vi "write module trace msg.vi"(8 "error in (no error)":errorcluster, 9 "Priority":T1(ring)=enum."Debug", 10 "message":string, 11 "module in":refnum<class "TBM module execution interface.lvclass">) -> (0 "error out":errorcluster, 3 "module out":refnum<class "TBM module execution interface.lvclass">)   [LabVIEW 2013, in "TBM module execution interface.lvclass"]
uses:
  TBM module execution interface.lvclass
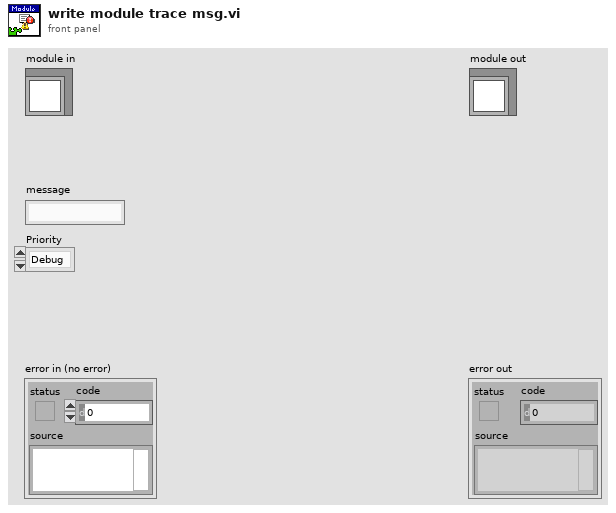
[diagram p1: front panel]
types:
  T1 = enum16{"Emergency", "Alert", "Critical", "Error", "Warning", "Notice", "Informational", "Debug"}
  T2 = enum16{"kern", "user", "mail", "daemon", "auth", "syslog", "lpr", "news", "uucp", "clk", "authpriv", "ftp", "NTP", "log audit", "log alert", "cron", "local0", "local1", "local2", "local3", "local4", "local5", "local6", "local7"}
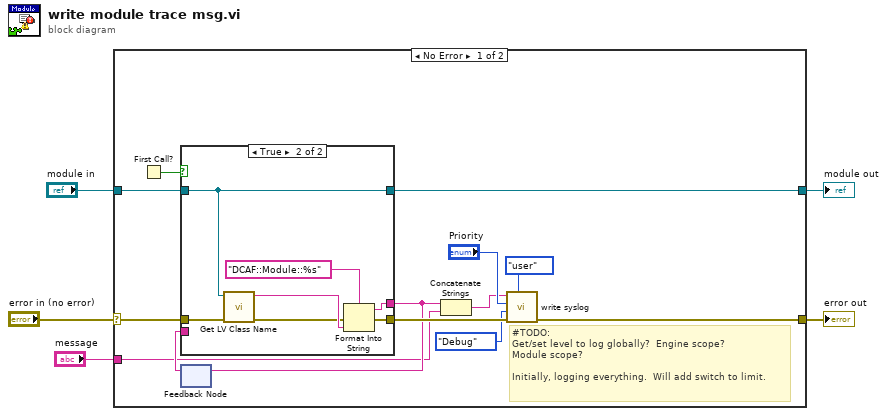
[diagram p0: block diagram]
diagram:
  n1 = case shown="No Error" "error in (no error)" {
    selector: "error in (no error)" -> [w14 w30]
    tunnel: [w12 w30] -> w4
    tunnel: [w16 w29] -> w2
    tunnel: "module in" -> [w17 w29]
    tunnel: "message" -> [w7 _]
    frame No Error {
      # "#TODO:\nGet/set level to log globally?  Engine scope?\nModule scope?\n\nInitially, logging everything.  Will add switch to limit."
      n2 = First Call?() -> (First Call?: T/F=w18:bool)
      n3 = feedback #1() -> (w15:string)  [unwired: 1 in]
      n4 = case shown="True" w18 {
        tunnel: w17 -> [w21 w28]
        tunnel: [w21 w28] -> w16
        tunnel: [w20 w22] -> w8
        tunnel: w15 -> [w20 _]
        tunnel: w14 -> [w19 w27]
        tunnel: [w19 w23] -> w13
        frame False {
        }
        frame True {
          n5 = call <vilib>:"Get LV Class Name.vi"("error in (no error)"=w27, "object"=w28) -> ("error out"=w24:errorcluster, "class name"=w25:string)  [unwired: 8 in]
          n6 = Format Into String(format string="DCAF::Module::%s", error in=w24, w25) -> (resulting string=w22:string, error out=w23:errorcluster)  [unwired: 1 in]
        }
      }
      n7 = feedback-in #1(w8) -> ()
      n8 = Concatenate Strings(w8, w7) -> (w6:string)
      n9 = call <vilib>:"write syslog.vi"("Facility"=T2."user", "error in (no error)"=w13, "Minimum level to log"=T1."Debug", "Priority"="Priority", "msg"=w6) -> ("error out"=w12:errorcluster)  [unwired: 6 in]
    }
    frame Error {
    }
  }
  "error out" <- w4
  "module out" <- w2
